vi "Actor Core.vi"(8 "error in":errorcluster, 11 "InterferometryUI in":refnum<class "InterferometryUI.lvclass">) -> (0 "error out":errorcluster, 3 "Actor out":refnum<class "Actor.lvclass">)   [LabVIEW 2023, in "InterferometryUI.lvlib" / "InterferometryUI.lvclass"]
doc: "(<B>Filename</B>: Actor Framework.lvlib:Actor.lvclass:Actor Core.vi)\n\nReceives messages to the actor, reacts to them, and initiates any error handling that may shut the actor down.\n\nDescendant classes may override this VI to append parallel tasks for the actor to complete while it handles messages. Overrides use the Call Parent Class Method node."
uses:
  InterferometryUI.lvclass
  ArduinoTranslationStageUI/ArduinoTranslationStageActor/ArduinoTranslationStage Messages/Init Msg/Init Msg.lvclass
  ConcreteClasses/ConcreteInstrumentClasses/CameraClasses/ZWO_ASI_LV/ZWO_ASI Messages/OpenCamera Msg/OpenCamera Msg.lvclass
  ArduinoTranslationStageUI/ArduinoTranslationStageActor/ArduinoTranslationStage Messages/MoveBySteps Msg/MoveBySteps Msg.lvclass
  <vilib>/ActorFramework/Stop Msg/Stop Msg.lvclass
  ConcreteClasses/ConcreteInstrumentClasses/CameraClasses/ZWO_ASI_LV/ZWO_ASI Messages/StopCapture Msg/StopCapture Msg.lvclass
  ConcreteClasses/ConcreteInstrumentClasses/CameraClasses/ZWO_ASI_LV/ZWO_ASI Messages/StartCapture Msg/StartCapture Msg.lvclass
  <vilib>/ActorFramework/Actor/Actor.lvclass
  ArduinoTranslationStageUI/ArduinoTranslationStageActor/ArduinoTranslationStage Actor/ArduinoTranslationStage.lvclass
  ConcreteClasses/ConcreteInstrumentClasses/CameraClasses/ZWO_ASI_LV/ZWO_ASI/ZWO_ASI.lvclass
  ConcreteClasses/ConcreteInstrumentClasses/CameraClasses/ZWO_ASI_LV/ZWO_ASI Messages/FindInstruments Msg/FindInstruments Msg.lvclass
  typedefs/instrumentType.ctl
  typedefs/typedefs.lvlib
  typedefs/InstrumentData.ctl
  ConcreteClasses/ConcreteInstrumentClasses/CameraClasses/ZWO_ASI_LV/ZWO_ASI Messages/SetExposure Msg/SetExposure Msg.lvclass
  C:/Program Files/National Instruments/LabVIEW 2023/vi.lib/ActorFramework/Actor/Actor.lvclass
  C:/Users/quantum/Documents/LVDAQ/UIs/InterferometryUI/InterferometryUI/InterferometryUI.lvclass
  C:/Users/quantum/Documents/LVDAQ/Interfaces/InitDeinitInterface/InitDeinitComm/InitDeinitComm.lvclass
  C:/Users/quantum/Documents/LVDAQ/Interfaces/AbstractInstrumentClasses/TranslationStages_LV/TranslationStagesComm/TranslationStagesComm.lvclass
  C:/Users/quantum/Documents/LVDAQ/UIs/ArduinoTranslationStageUI/ArduinoTranslationStageActor/ArduinoTranslationStage Actor/ArduinoTranslationStage.lvclass
  C:/Users/quantum/Documents/LVDAQ/Interfaces/InitDeinitInterface/InitDeinit/InitDeinit.lvclass
  C:/Users/quantum/Documents/LVDAQ/Interfaces/AbstractInstrumentClasses/StepperMotorControllers_LV/StepperMotorController/StepperMotorController.lvclass
  C:/Users/quantum/Documents/LVDAQ/Interfaces/AbstractInstrumentClasses/TranslationStages_LV/TranslationStageInterface/TranslationStagesInterface.lvclass
  C:/Users/quantum/Documents/LVDAQ/ConcreteClasses/ConcreteInstrumentClasses/CameraClasses/ZWO_ASI_LV/ZWO_ASI/ZWO_ASI.lvclass
  C:/Users/quantum/Documents/LVDAQ/Interfaces/AbstractInstrumentClasses/Cameras_LV/CameraInterface/CameraInterface.lvclass
  InterferometryUIPublicData.ctl
panel:
  in  "input cluster":T1={"Scanning Segments Left"=0, "Scanning"=FALSE, "Path"=path "", "FileName"="", "Scan Segments"=0, "Step Time (us)"=100, "Polarity"=enum."Positive", "Direction"=enum."Forward", "Steps"=1, "Image"=[]} {"Steps" min=1 max=10000 step=1 scale=1.0..10000.0; "Step Time (us)" min=100 step=10 scale=100.0..10000.0; "Scan Segments" max=100 step=1 scale=0.0..100.0}
  in  "Find Cameras":bool
  in  "FileName":string
  in  "Path":path
  in  "Exposure (ms)":u32
  out "VI":refnum<vi>
  out "Image":u16[][](graph)
  in  "Snap":bool
  in  "Live":bool
  in  "Stop Button":bool
  in  "Scan":bool
  in  "Move Stepper":bool
  in  "Connect Cam":bool
  in  "Connect Stepper":bool
  in  "VISA resource name":refnum<visa-resource-name>
  in  "Direction":enum16{"Forward", "Backwards"}(ring)
  in  "Polarity":enum16{"Positive", "Negative"}(ring)=enum."Negative"
  in  "Step Time (us)":u32(slide)=100 min=100 step=10 scale=100.0..10000.0
  in  "Steps":u32(slide)=1 min=1 max=10000 step=1 scale=1.0..10000.0
  in  "Scan Segments":u32(slide) max=100 step=1 scale=0.0..100.0
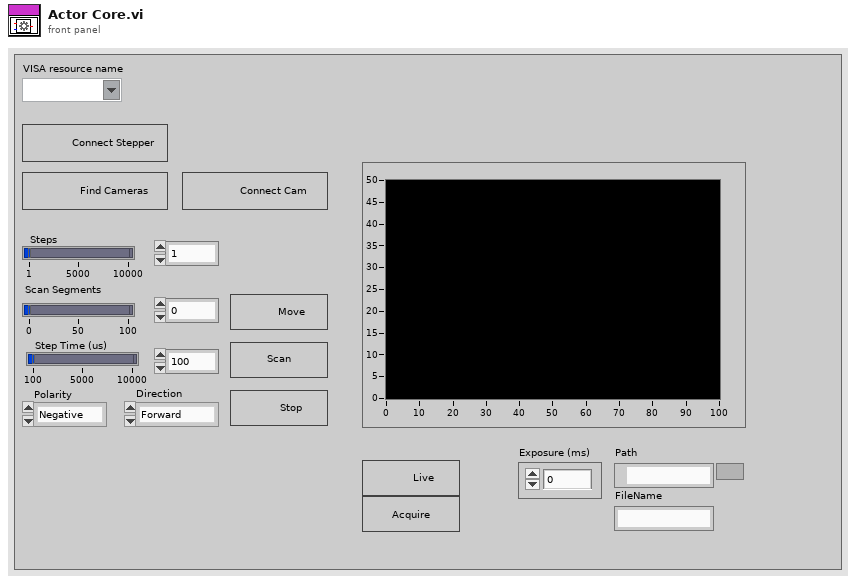
[diagram p1: front panel]
types:
  T1 = typedef "InterferometryUIPublicData.ctl" = cluster{"Scanning Segments Left":u16, "Scanning":bool, "Path":path, "FileName":string, "Scan Segments":u32, "Step Time (us)":u32, "Polarity":enum16{"Positive", "Negative"}, "Direction":enum16{"Forward", "Backwards"}, "Steps":u32, "Image":u16[][]}
  T2 = typedef "typedefs.lvlib/InstrumentData.ctl" = cluster{"Instr Error":errorcluster, "Address":cluster{"address type":enum16{"VISA", "Index"}, "Address":string, "instrument type":T3}, "CurrentState":cluster{"Initialized":bool, "Connected":bool, "Running":bool, "Error":bool}}
  T3 = typedef "typedefs.lvlib/instrumentType.ctl" = enum16{"Spectrometer", "Camera", "Stepper", "Piezo", "SLM"}
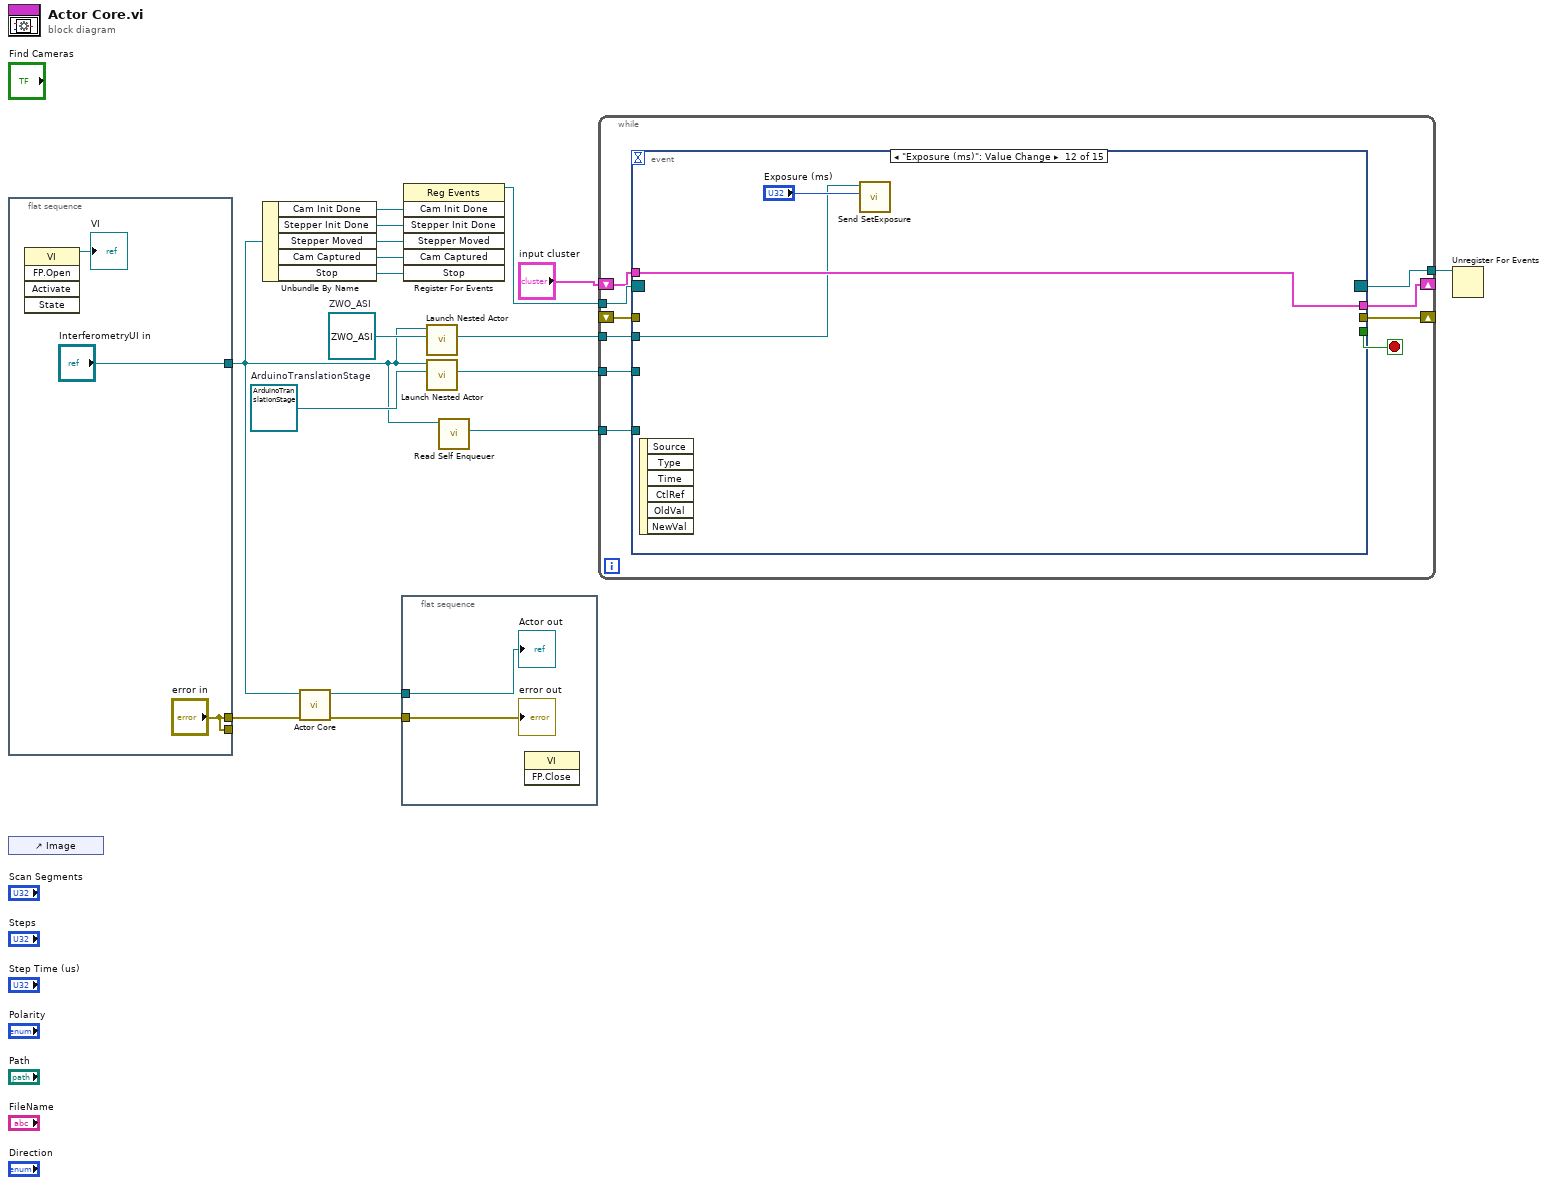
[diagram p0: block diagram]
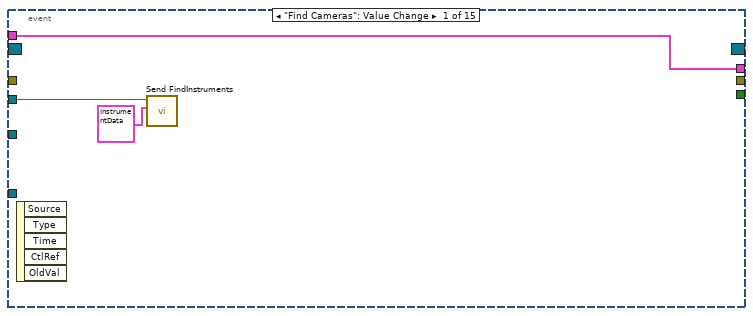
[diagram p2: hidden frame]
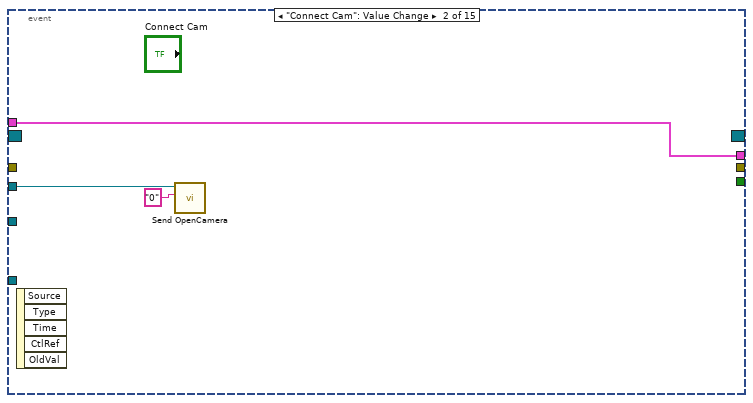
[diagram p3: hidden frame]
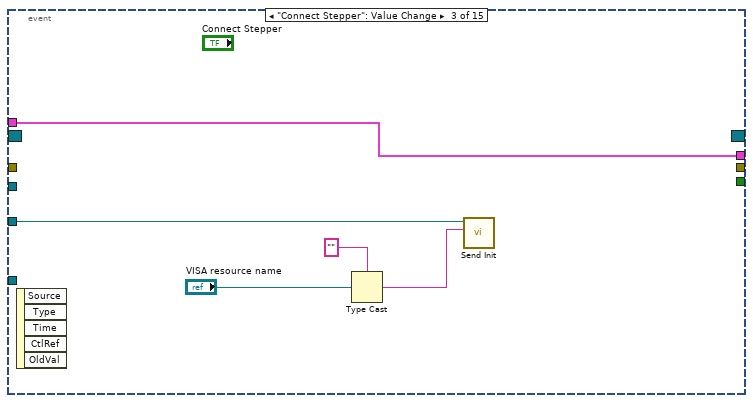
[diagram p4: hidden frame]
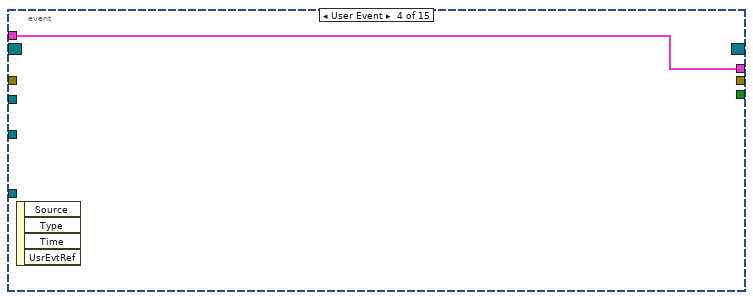
[diagram p5: hidden frame]
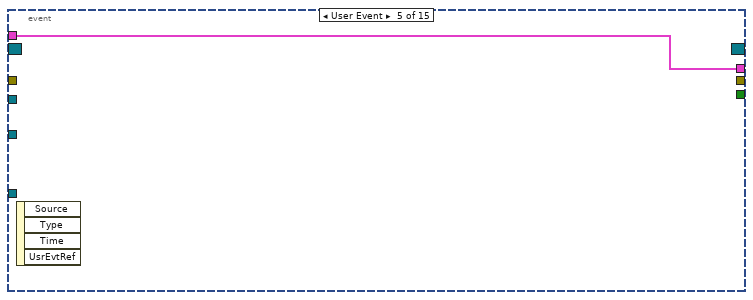
[diagram p6: hidden frame]
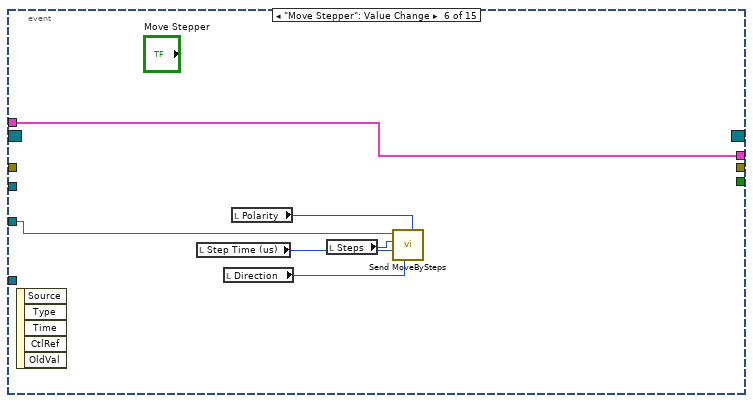
[diagram p7: hidden frame]
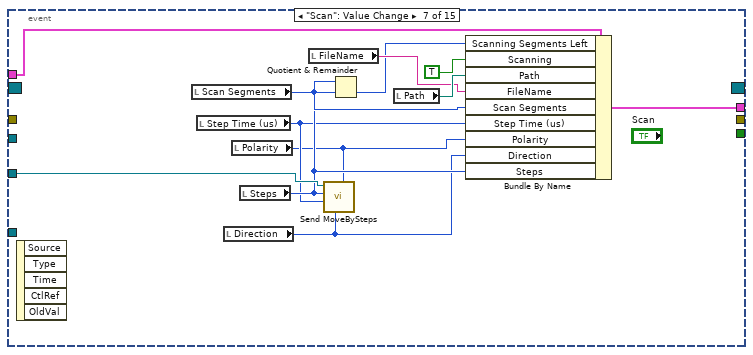
[diagram p8: hidden frame]
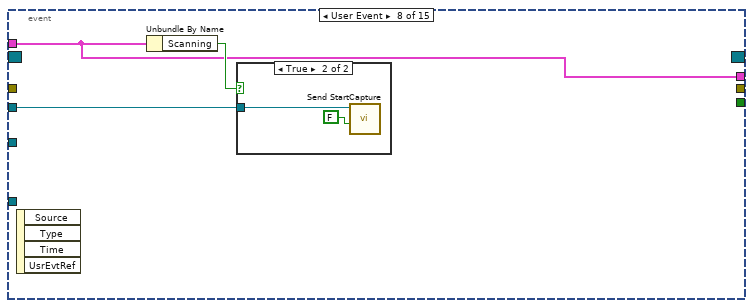
[diagram p9: hidden frame]
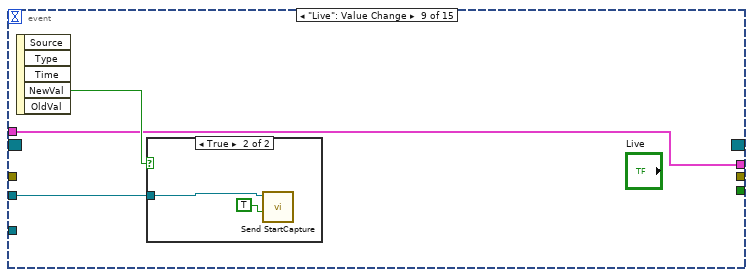
[diagram p11: hidden frame]
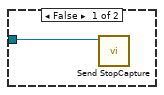
[diagram p12: hidden frame]
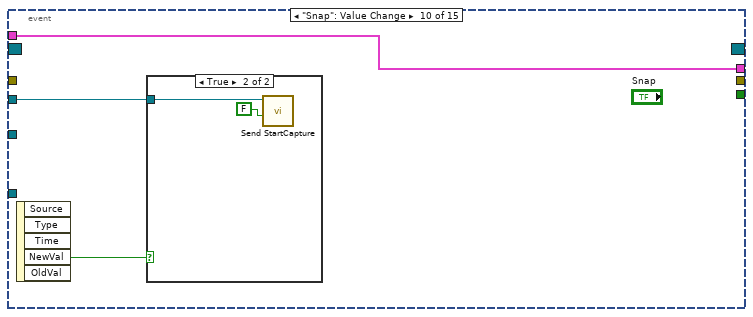
[diagram p13: hidden frame]
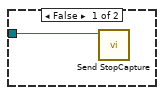
[diagram p14: hidden frame]
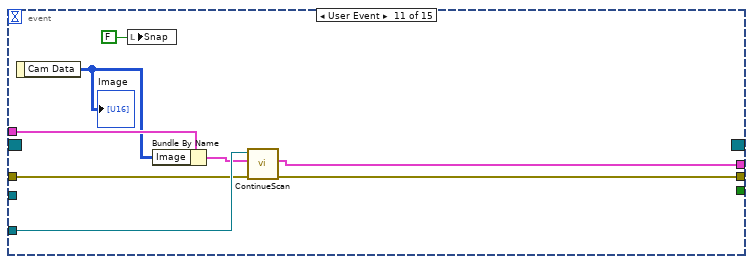
[diagram p15: hidden frame]
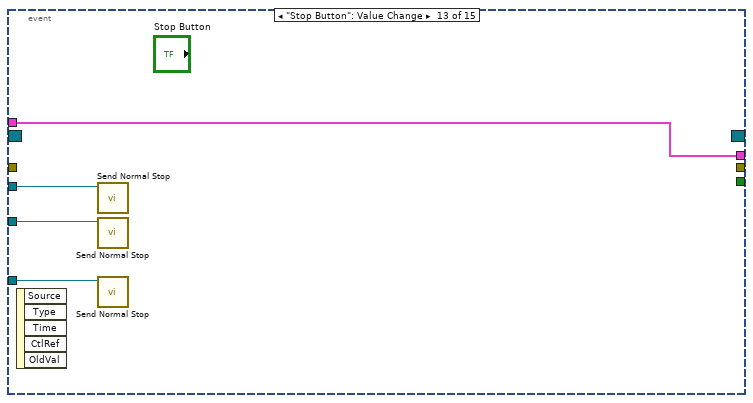
[diagram p16: hidden frame]
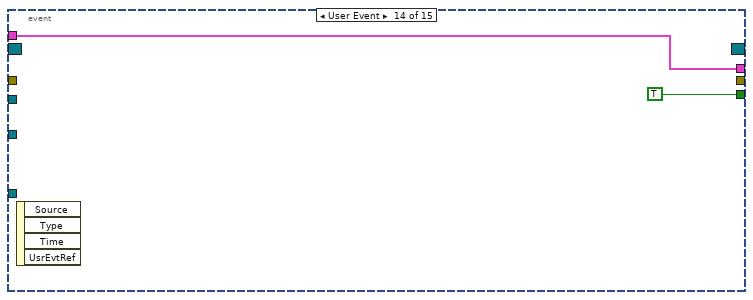
[diagram p17: hidden frame]
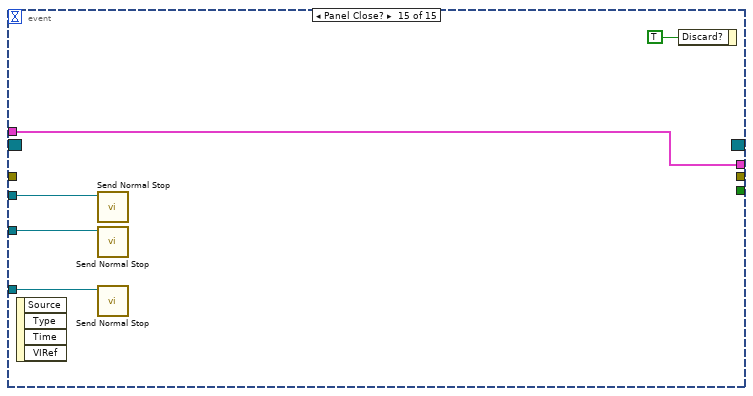
[diagram p18: hidden frame]
diagram:
  w12 = refnum<class "ZWO_ASI.lvclass"> refnum  # ZWO_ASI
  w13 = refnum<class "ArduinoTranslationStage.lvclass"> refnum  # ArduinoTranslationStage
  n1 = flat-sequence {
    tunnel: ["error in"] -> w5
    tunnel: ["InterferometryUI in"] -> w3
    tunnel: ["error in"] -> _
    frame #0 {
      n2 = invoke class="VI" method="FP.Open"() -> (reference out=→"VI":refnum<vi>)  [unwired: 5 in, 4 out]
    }
  }
  n3 = control-ref of="Image"() -> ()  [unwired: 1 out]
  n4 = Unbundle By Name(w3) -> ("Cam Init Done"=w10:refnum<user-event>, "Stepper Init Done"=w9:refnum<user-event>, "Stepper Moved"=w8:refnum<user-event>, "Cam Captured"=w7:refnum<user-event>, "Stop"=w6:refnum<user-event>)
  n5 = call-parent "Actor Core.vi"("error in"=w5, "Actor in"=w3) -> ("error out"=w17:errorcluster, "Actor out"=w4:refnum<class "Actor.lvclass">)  [unwired: 8 in]
  n6 = flat-sequence {
    tunnel: w17 -> [w22]
    tunnel: w4 -> [w21]
    frame #0 {
      n7 = invoke class="VI" method="FP.Close"() -> ()  [unwired: 3 in, 3 out]
      "error out" <- w22
      "Actor out" <- w21
    }
  }
  n8 = register-events(w10, w9, w8, w7, w6) -> (reference out=w11:refnum<event-registration>)  [unwired: 2 in, 1 out]
  n9 = call <vilib>:"Launch Nested Actor.vi"("Nested Actor"=w12, "Caller Actor in"=w3) -> ("Nested Actor's Enqueuer"=w14:refnum<class "Message Enqueuer.lvclass">)  [unwired: 7 in, 2 out]
  n10 = call <vilib>:"Launch Nested Actor.vi"("Nested Actor"=w13, "Caller Actor in"=w3) -> ("Nested Actor's Enqueuer"=w16:refnum<class "Message Enqueuer.lvclass">)  [unwired: 7 in, 2 out]
  n11 = call <vilib>:"Read Self Enqueuer.vi"("Actor"=w3) -> ("Self Enqueuer"=w15:refnum<class "Message Enqueuer.lvclass">)  [unwired: 10 in]
  n12 = while {
    tunnel: w16 -> [w31]
    tunnel: w15 -> [w32]
    tunnel: w14 -> [w28]
    tunnel: w11 -> [w30]
    tunnel: [w27] -> w2
    shift-right: [w25] -> _
    shift-left: "input cluster" -> [w26]
    shift-right: [w24] -> _
    shift-left: _ -> [w23]
    stop <- w29 stop-if-true
    n13 = event shown="[11] \"Exposure (ms)\": Value Change" {
      selector: w30 -> [_ _ _ _ _ _ _ _ _ _ _ _ _ _ _]
      dyn-events: [_ _ _ _ _ _ _ _ _ _ _ _ _ _ _] -> w27
      timeout: _ -> [_ _ _ _ _ _ _ _ _ _ _ _ _ _ _]
      tunnel: w32 -> [_ _ _ _ _ _ _ _ _ _ _ _ w95 _ w102]
      tunnel: w31 -> [_ _ w41 _ _ w46 w63 _ _ _ w88 _ w94 _ w100]
      tunnel: [_ _ _ _ _ _ _ _ _ _ _ _ _ TRUE _] -> w29
      tunnel: w28 -> [w35 w38 _ _ _ _ _ w66 w71 w77 _ w89 w93 _ w99]
      tunnel: w26 -> [w33 w36 w39 w44 w45 w47 w59 w64 w69 w75 w85 w91 w92 w96 w98]
      tunnel: [w33 w36 w39 w44 w45 w47 w60 w64 w69 w75 w87 w91 w92 w96 w98] -> w25
      tunnel: [_ _ _ _ _ _ _ _ _ _ w82 _ _ _ _] -> w24
      tunnel: w23 -> [_ _ _ _ _ _ _ _ _ _ w81 _ _ _ _]
      event "Find Cameras": Value Change {
        n14 = event-data() -> ()  [unwired: 1 in, 5 out]
        n15 = call "Send FindInstruments.vi"("InstrumentData"=T2 {"Instr Error"={"status"=FALSE, "code"=0, "source"=""}, "Address"={"address type"=enum."VISA", "Address"="", "instrument type"=enum."Spectrometer"}, "CurrentState"={"Initialized"=FALSE, "Connected"=FALSE, "Running"=FALSE, "Error"=FALSE}}, "Message Enqueuer"=w35) -> ()  [unwired: 8 in, 2 out]
      }
      event "Connect Cam": Value Change {
        n16 = event-data() -> ()  [unwired: 1 in, 5 out]
        n17 = call "Send OpenCamera.vi"("Camera ID"="0", "Message Enqueuer"=w38) -> ()  [unwired: 8 in, 2 out]
      }
      event "Connect Stepper": Value Change {
        n18 = event-data() -> ()  [unwired: 1 in, 5 out]
        n19 = Type Cast(type="", x="VISA resource name") -> (*(type *) &x=w40:string)
        n20 = call "Send Init.vi"("Address"=w40, "Message Enqueuer"=w41) -> ()  [unwired: 8 in, 2 out]
      }
      event User Event {
        n21 = event-data() -> ()  [unwired: 1 in, 4 out]
      }
      event User Event {
        n22 = event-data() -> ()  [unwired: 1 in, 4 out]
      }
      event "Move Stepper": Value Change {
        n23 = event-data() -> ()  [unwired: 1 in, 5 out]
        n24 = local read "Step Time (us)"() -> (w50:u32)
        n25 = local read "Direction"() -> (w48:enum16{"Forward", "Backwards"})
        n26 = local read "Polarity"() -> (w49:enum16{"Positive", "Negative"})
        n27 = local read "Steps"() -> (w51:u32)
        n28 = call "Send MoveBySteps.vi"("Polarity"=w49, "Direction"=w48, "Speed"=w50, "Steps"=w51, "Message Enqueuer"=w46) -> ()  [unwired: 5 in, 2 out]
      }
      event "Scan": Value Change {
        n29 = event-data() -> ()  [unwired: 1 in, 5 out]
        n30 = local read "Scan Segments"() -> (w56:u32)
        n31 = local read "Step Time (us)"() -> (w54:u32)
        n32 = local read "Direction"() -> (w53:enum16{"Forward", "Backwards"})
        n33 = local read "Polarity"() -> (w52:enum16{"Positive", "Negative"})
        n34 = local read "Steps"() -> (w55:u32)
        n35 = local read "FileName"() -> (w61:string)
        n36 = call "Send MoveBySteps.vi"("Polarity"=w52, "Direction"=w53, "Speed"=w54, "Steps"=w55, "Message Enqueuer"=w63) -> ()  [unwired: 5 in, 2 out]
        n37 = Quotient & Remainder(x=w55, y=w56) -> (floor(x/y)=w58:u32)  [unwired: 1 out]
        n38 = local read "Path"() -> (w62:path)
        n39 = Bundle By Name(cluster=w59, "Scanning Segments Left"=w58, "Scanning"=TRUE, "Path"=w62, "FileName"=w61, "Scan Segments"=w56, "Step Time (us)"=w54, "Polarity"=w52, "Direction"=w53, "Steps"=w55) -> (w60:T1)
      }
      event User Event {
        n40 = event-data() -> ()  [unwired: 1 in, 4 out]
        n41 = Unbundle By Name(w64) -> ("Scanning"=w65:bool)
        n42 = case shown="True" w65 {
          tunnel: w66 -> [_ w68]
          frame False {
          }
          frame True {
            n43 = call "Send StartCapture.vi"("Continuous"=FALSE, "Message Enqueuer"=w68) -> ()  [unwired: 8 in, 2 out]
          }
        }
      }
      event "Live": Value Change {
        n44 = event-data() -> ("NewVal"=w70:bool)  [unwired: 1 in, 4 out]
        n45 = case shown="True" w70 {
          tunnel: w71 -> [w72 w74]
          frame False {
            n46 = call "Send StopCapture.vi"("Message Enqueuer"=w72) -> ()  [unwired: 9 in, 2 out]
          }
          frame True {
            n47 = call "Send StartCapture.vi"("Continuous"=TRUE, "Message Enqueuer"=w74) -> ()  [unwired: 8 in, 2 out]
          }
        }
      }
      event "Snap": Value Change {
        n48 = event-data() -> ("NewVal"=w76:bool)  [unwired: 1 in, 4 out]
        n49 = case shown="True" w76 {
          tunnel: w77 -> [w78 w80]
          frame False {
            n50 = call "Send StopCapture.vi"("Message Enqueuer"=w78) -> ()  [unwired: 9 in, 2 out]
          }
          frame True {
            n51 = call "Send StartCapture.vi"("Continuous"=FALSE, "Message Enqueuer"=w80) -> ()  [unwired: 8 in, 2 out]
          }
        }
      }
      event User Event {
        n52 = event-data() -> ("Cam Data"=w84:u16[][])  [unwired: 1 in]
        "Image" <- w84
        n53 = local write "Snap"(FALSE ("Snap")) -> ()
        n54 = Bundle By Name(cluster=w85, "Image"=w84) -> (w83:T1)
        n55 = call "ContinueScan.vi"("error in"=w81, "input cluster"=w83, "Message Enqueuer in"=w88) -> ("error out"=w82:errorcluster, "output cluster"=w87:T1)  [unwired: 7 in]
      }
      event "Exposure (ms)": Value Change {
        n56 = event-data() -> ()  [unwired: 1 in, 6 out]
        n57 = call "Send SetExposure.vi"("Exposure(ms)"="Exposure (ms)", "Message Enqueuer"=w89) -> ()  [unwired: 8 in, 2 out]
      }
      event "Stop Button": Value Change {
        n58 = event-data() -> ()  [unwired: 1 in, 5 out]
        n59 = call <vilib>:"Send Normal Stop.vi"("Message Enqueuer"=w93) -> ()  [unwired: 10 in, 1 out]
        n60 = call <vilib>:"Send Normal Stop.vi"("Message Enqueuer"=w94) -> ()  [unwired: 10 in, 1 out]
        n61 = call <vilib>:"Send Normal Stop.vi"("Message Enqueuer"=w95) -> ()  [unwired: 10 in, 1 out]
      }
      event User Event {
        n62 = event-data() -> ()  [unwired: 1 in, 4 out]
      }
      event Panel Close? {
        n63 = event-data() -> ()  [unwired: 1 in, 4 out]
        n64 = call <vilib>:"Send Normal Stop.vi"("Message Enqueuer"=w99) -> ()  [unwired: 10 in, 1 out]
        n65 = call <vilib>:"Send Normal Stop.vi"("Message Enqueuer"=w100) -> ()  [unwired: 10 in, 1 out]
        n66 = call <vilib>:"Send Normal Stop.vi"("Message Enqueuer"=w102) -> ()  [unwired: 10 in, 1 out]
        n67 = event-data("Discard?"=TRUE) -> ()  [unwired: 1 in, 1 out]
      }
    }
  }
  n68 = Unregister For Events(event registration refnum=w2) -> ()  [unwired: 1 in, 1 out]
